vi "SVPO Analog Tacho Process (1 Ch DBL Array) with IC.vi"(0 "analog tacho signal":dbl[](array[numeric]), 1 "initial conditions":T1, 2 "reset? (F)":bool, 5 "sampling rate [Hz]":dbl=1.0, 7 "threshold":dbl format="%.2f", 9 "pulse/revolution (1)":i32=1, 11 "hysteresis (0)":dbl format="%.2f", 12 "pulse width (2)":i32=2, 13 "slope (Rising)":u16(ring) items=["Rising", "Falling"]) -> (3 "final conditions":T1, 4 "speed position info":T2, 6 "current speed [RPM]":dbl)   [LabVIEW 2017, in "SoundVib_TachProcess.lvlib"]
doc: "Locates tachometer pulse positions in analog tachometer signals using the number of generated pulses per revolution, the pulse width, and the arrival edge of the tachometer pulse. Use this VI on embedded targets that have limited computational resources. Wire data to the <B>analog tacho signal</B> input to determine the polymorphic instance to use or manually select the instance."
uses:
  <vilib>/addons/Sound and Vibration/Order Analysis/Tach Process/SoundVib_TachProcess.lvlib
  <vilib>/addons/Sound and Vibration/Order Analysis/Misc/OAT Position Info.ctl
  <vilib>/addons/_NISVFA/_Shared subVIs/Controls/svc_Analog Tacho State.ctl
  <vilib>/addons/_NISVFA/_Shared subVIs/Common/SV Buffer Array (No State) (DBL).vi
  <vilib>/addons/Sound and Vibration/Order Analysis/Tach Process/SubVIs/OAT Cross Point Detection.vi
  <vilib>/addons/_NISVFA/_Shared subVIs/Common/svc_Get Array Subset (Index).vi
  <vilib>/Analysis/8numeric.llb/Threshold Detector.vi
  <vilib>/addons/_NISVFA/_Shared subVIs/Common/svc_Coerce Index and Length.vi
  <vilib>/addons/_NISVFA/_Shared subVIs/Common/svc_Conditional Merge Error.vi
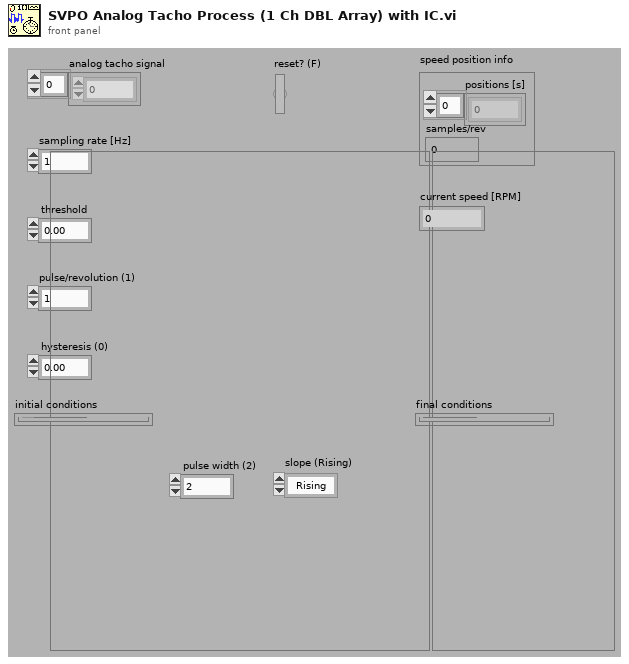
[diagram p1: front panel]
types:
  T1 = typedef "svc_Analog Tacho State.ctl" = cluster{"hysteresis state":dbl, "edge detection state":cluster{"x[n]":dbl[], "size":dbl}, "pulse to speed state":cluster{"pulse positions":dbl[], "elapsed time":dbl}}
  T2 = typedef "OAT Position Info.ctl" = cluster{"positions [s]":dbl[], "samples/rev":dbl}
  T3 = cluster{"pulse positions":dbl[], "elapsed time":dbl}
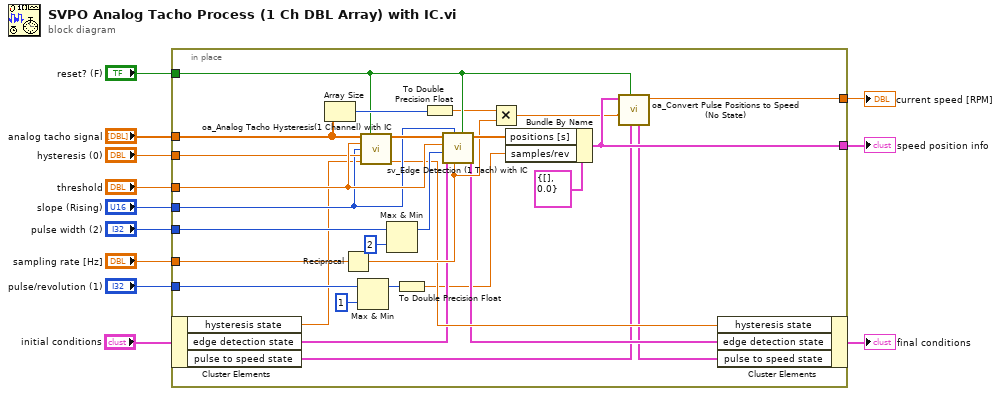
[diagram p0: block diagram]
diagram:
  n1 = in-place {
    in-place-border: "threshold" -> [w40]
    in-place-border: "pulse/revolution (1)" -> [w39]
    in-place-border: "hysteresis (0)" -> [w35]
    in-place-border: "pulse width (2)" -> [w33]
    in-place-border: "sampling rate [Hz]" -> [w30]
    in-place-border: "analog tacho signal" -> [w28]
    in-place-border: "reset? (F)" -> [w25]
    in-place-border: [w24] -> w5
    in-place-border: [w23] -> w4
    in-place-border: "slope (Rising)" -> [w21]
    n2 = in-place-cluster #1("initial conditions") -> ("hysteresis state"=w20:dbl, "edge detection state"=w18:cluster{"x[n]":dbl[], "size":dbl}, "pulse to speed state"=w16:T3)
    n3 = Array Size(array=w28) -> (size(s)=w27:i32)
    n4 = Reciprocal(x=w30) -> (1/x=w26:dbl)
    n5 = Max & Min(x=w39, y=1) -> (max(x,y)=w37:i32)  [unwired: 1 out]
    n6 = call <vilib>:"oa_Analog Tacho Hysteresis(1 Channel) with IC.vi"("input signal"=w28, "reset? (T)"=w25, "threshold (auto)"=w40, "slope (Rising)"=w21, "hysteresis(0)"=w35, "initial condition"=w20) -> ("output signal"=w36:dbl[], "final condition"=w19:dbl)  [unwired: 8 in]
    n7 = Max & Min(x=w33, y=2) -> (max(x,y)=w34:i32)  [unwired: 1 out]
    n8 = To Double Precision Float(number=w37) -> (double precision float=w13:dbl)
    n9 = To Double Precision Float(number=w27) -> (double precision float=w14:dbl)
    n10 = call <vilib>:"sv_Edge Detection (1 Tach) with IC.vi"("reset? (True)"=w25, "dt"=w26, "slope (Rising)"=w21, "initial conditions"=w18, "pulse width (2)"=w34, "threshold (0.0)"=w40, "x[n]"=w36) -> ("final conditions"=w17:cluster{"x[n]":dbl[], "size":dbl}, "pulse positions [s]"=w31:dbl[])  [unwired: 3 in]
    n11 = Multiply(x=w14, y=w26) -> (x*y=w22:dbl)
    n12 = Bundle By Name(cluster=T2 {"positions [s]"=[], "samples/rev"=0.0} ("speed position info"), "positions [s]"=w31, "samples/rev"=w13) -> (w24:T2)
    n13 = call <vilib>:"oa_Convert Pulse Positions to Speed (No State).vi"("state in"=w16, "reset?"=w25, "waveform duration"=w22, "speed position info"=w24) -> ("speed [RPM]"=w23:dbl, "state out"=w15:T3)  [unwired: 6 in]
    n14 = in-place-cluster #1("hysteresis state"=w19, "edge detection state"=w17, "pulse to speed state"=w15) -> (→"final conditions":T1)
  }
  "speed position info" <- w5
  "current speed [RPM]" <- w4
